vi "ROW AND COLUMN.vi"() -> ()   [LabVIEW 2019]
panel:
  out "column":dbl[](array[numeric])
  out "ROW":dbl[](array[numeric])
  in  "2-DIMENSIONAL ARRAY":dbl[][](array[numeric])=[[10.0, 20.0, 30.0], [40.0, 50.0, 60.0], [70.0, 80.0, 90.0]]
  out "element 2":dbl
  out "element":dbl
  in  "ONE DIMENSIONAL ARRAY":dbl[](array[numeric])=[10.0, 20.0, 30.0, 40.0, 50.0]
  # "INDEX ARRAY"
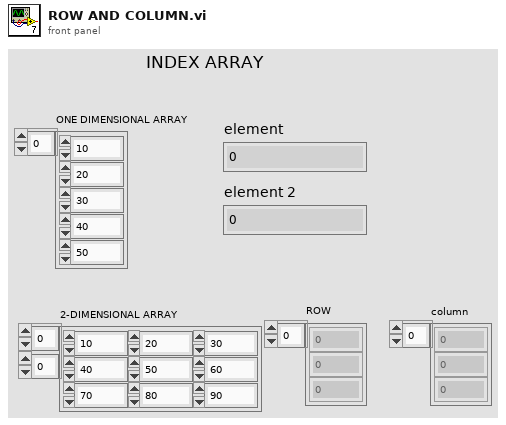
[diagram p1: front panel]
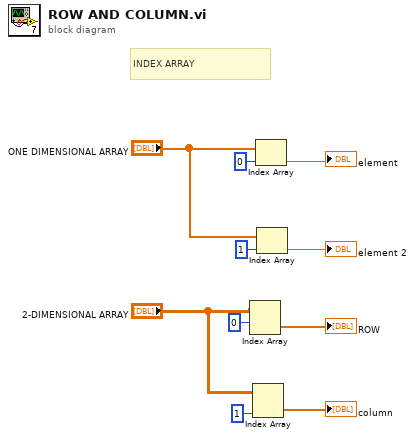
[diagram p0: block diagram]
diagram:
  # "INDEX ARRAY"
  n1 = Index Array(array="2-DIMENSIONAL ARRAY", index (row)=0) -> (element=→"ROW":dbl[])  [unwired: 1 in]
  n2 = Index Array(array="2-DIMENSIONAL ARRAY", index (col)=1 ("disabled index (col)")) -> (element=→"column":dbl[])  [unwired: 1 in]
  n3 = Index Array(array="ONE DIMENSIONAL ARRAY", index=0) -> (element=→"element":dbl)
  n4 = Index Array(array="ONE DIMENSIONAL ARRAY", index=1) -> (element=→"element 2":dbl)
